vi "HC-SR 04 read.vi"(8 "error in (no error)":errorcluster, 11 "I2C Ref Out in":T1) -> (0 "error out":errorcluster, 1 "Right":dbl, 2 "Left":dbl, 3 "I2C Ref Out out":T1, 5 "32bit integer":i32[](array[numeric]))   [LabVIEW 2019]
uses:
  <vilib>/myRIO/Instrument Drivers/Onboard IO/I2C/typedefs/I2C Reference.ctl
  <vilib>/myRIO/Common/Instrument Driver Framework/Utilities/typedefs/myRIO Generic Hardware Reference.ctl
  <vilib>/myRIO/Common/Instrument Driver Framework/Utilities/typedefs/Hardware Version Enum.ctl
  <vilib>/myRIO/Common/Instrument Driver Framework/Utilities/typedefs/myRIO v1.0 Reference.ctl
  <vilib>/myRIO/Common/Instrument Driver Framework/Utilities/typedefs/Generic FPGA Reference.ctl
  <vilib>/myRIO/Common/Instrument Driver Framework/myRIO v1.0/I2C/typedefs/I2C Channels Enum.ctl
  <vilib>/myRIO/Instrument Drivers/Onboard IO/I2C/typedefs/I2C Configuration.ctl
  <vilib>/myRIO/Instrument Drivers/Onboard IO/I2C/typedefs/I2C Transfer Rate.ctl
  <vilib>/Utility/error.llb/Error Cluster From Error Code.vi
  <vilib>/myRIO/Common/Instrument Driver Framework/myRIO v1.0/I2C/vis/myRIO v1.0 Read I2C.vi
  <vilib>/myRIO/Instrument Drivers/Onboard IO/I2C/I2C.lvlib
  <vilib>/ptbypt/NI_PtbyPt.lvlib
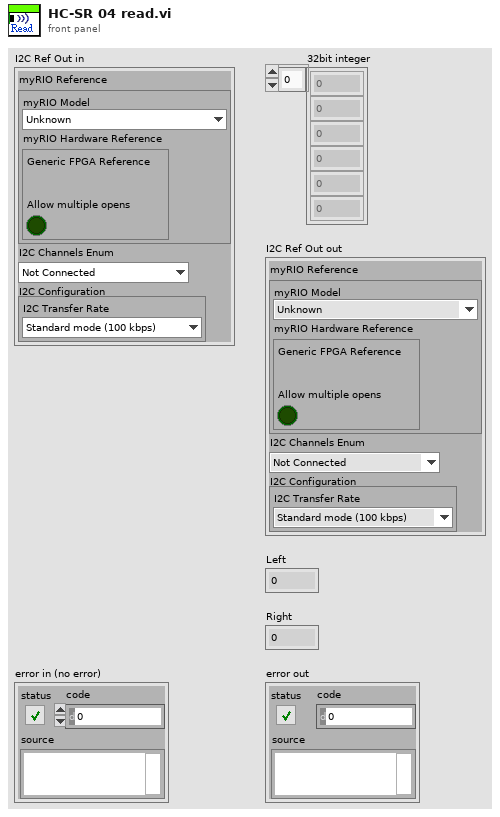
[diagram p1: front panel]
types:
  T1 = typedef "I2C.lvlib/I2C Reference.ctl" = cluster{"myRIO Reference":T2, "I2C Channels Enum":T6, "I2C Configuration":T7}
  T2 = typedef "myRIO Generic Hardware Reference.ctl" = cluster{"myRIO Model":T3, "myRIO Hardware Reference":T4}
  T3 = typedef "Hardware Version Enum.ctl" = enum16{"Unknown", "myRIO-1900", "myRIO-1950", "roboRIO", "NI ELVIS RIO CM", "ELVIS III"}
  T4 = typedef "myRIO v1.0 Reference.ctl" = cluster{"Generic FPGA Reference":T5, "Allow multiple opens":bool}
  T5 = typedef "Generic FPGA Reference.ctl" = refnum<k20>
  T6 = typedef "I2C Channels Enum.ctl" = enum16{"Not Connected", "A/I2C", "B/I2C", "I2C/I2C"}
  T7 = typedef "I2C.lvlib/I2C Configuration.ctl" = cluster{"I2C Transfer Rate":T8}
  T8 = typedef "I2C.lvlib/I2C Transfer Rate.ctl" = enum16{"Standard mode (100 kbps)", "Fast mode (400 kbps)"}
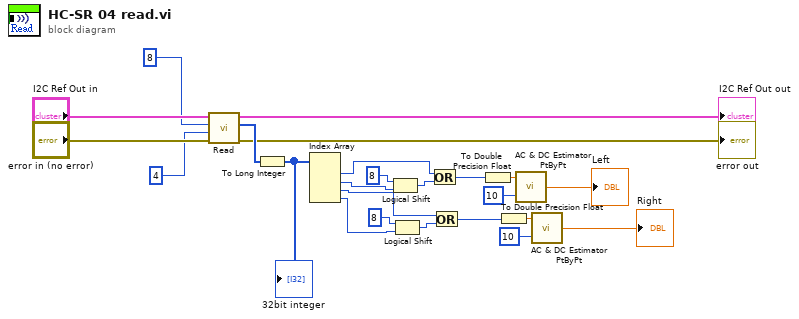
[diagram p0: block diagram]
diagram:
  n1 = call <vilib>:"Read.vi"("error in (no error)"="error in (no error)", "Byte Count"=u32 4, "Slave Address (7-bit)"=u8 8, "I2C Ref In"="I2C Ref Out in") -> ("error out"=→"error out":errorcluster, "Bytes Read"=w15:u8[], "I2C Ref Out"=→"I2C Ref Out out":T1)  [unwired: 4 in]
  n2 = To Long Integer(number=w15) -> (32bit integer=w16:i32[])
  "32bit integer" <- w16
  n3 = Index Array(array=w16) -> (element #1=w20:i32, element #2=w18:i32, element #3=w23:i32, element #4=w24:i32)  [unwired: 4 in]
  n4 = Logical Shift(y=i16 8 ("x"), x=w18) -> (x << y=w19:i32)
  n5 = Logical Shift(y=i16 8 ("x"), x=w24) -> (x << y=w21:i32)
  n6 = Or(x=w20, y=w19) -> (x .or. y?=w8:i32)
  n7 = Or(x=w23, y=w21) -> (x .or. y?=w2:i32)
  n8 = To Double Precision Float(number=w8) -> (double precision float=w6:dbl)
  n9 = To Double Precision Float(number=w2) -> (double precision float=w3:dbl)
  n10 = call <vilib>:"AC & DC Estimator PtByPt.vi"("signal"=w6, "sample length"=10) -> ("DC estimate (V)"=→"Left":dbl)  [unwired: 1 in, 2 out]
  n11 = call <vilib>:"AC & DC Estimator PtByPt.vi"("signal"=w3, "sample length"=10) -> ("DC estimate (V)"=→"Right":dbl)  [unwired: 1 in, 2 out]
